vi "FinalizeHWI.vi"(8 "error in (no error)":errorcluster, 10 "Master Device in":refnum<class "Master Device.lvclass">, 11 "SRS_DS345 in":refnum<class "SRS_DS345.lvclass">) -> (0 "error out":errorcluster, 2 "Master Device out":refnum<class "Master Device.lvclass">, 3 "SRS_DS345 out":refnum<class "SRS_DS345.lvclass">)   [LabVIEW 2013, in "SRS_DS345.lvclass"]
uses:
  SRS_DS345.lvclass
  <vilib>/Utility/error.llb/DialogType.ctl
  Master Device/Master Device.lvclass
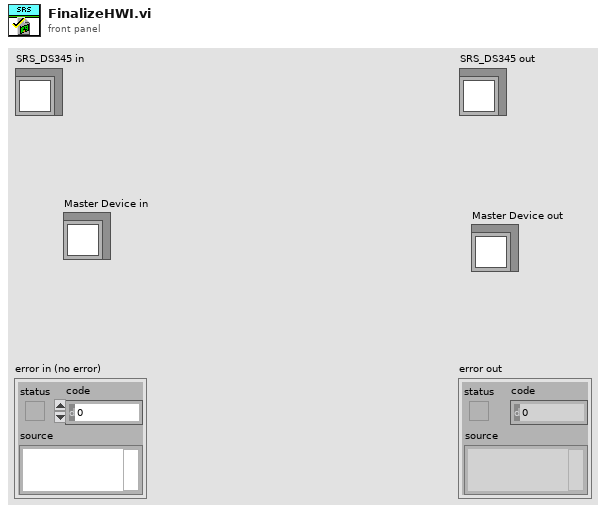
[diagram p1: front panel]
types:
  T1 = typedef "DialogType.ctl" = u16
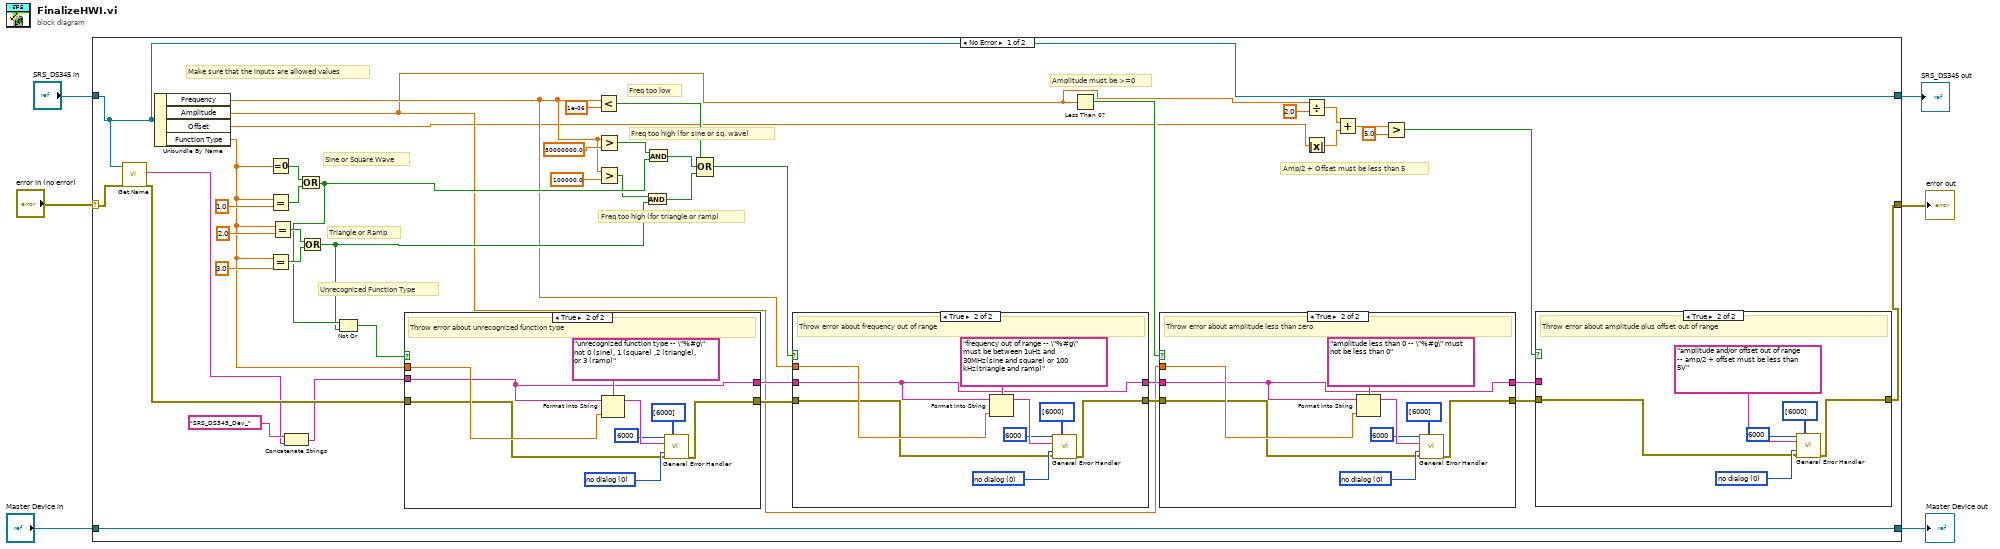
[diagram p0: block diagram]
diagram:
  n1 = case shown="No Error" "error in (no error)" {
    selector: "error in (no error)" -> [w42 w93]
    tunnel: [w8 w93] -> w5
    tunnel: [w9 w92] -> w3
    tunnel: "Master Device in" -> [w9 w92]
    tunnel: "SRS_DS345 in" -> [w7 w91]
    tunnel: [w7 w91] -> w1
    frame No Error {
      # "Amp/2 + Offset must be less than 5"
      # "Amplitude must be >=0"
      # "Freq too high (for triangle or ramp)"
      # "Freq too high (for sine or sq. wave)"
      # "Freq too low"
      # "Unrecognized Function Type"
      # "Triangle or Ramp"
      # "Sine or Square Wave"
      # "Make sure that the inputs are allowed values"
      n2 = call-dynamic "Get Name.vi"("error in (no error)"=w42, "Device in"=w7) -> ("error out"=w41:errorcluster, "Name"=w26:string)  [unwired: 7 in, 1 out]
      n3 = Unbundle By Name(w7) -> ("Frequency"=w23:dbl, "Amplitude"=w19:dbl, "Offset"=w17:dbl, "Function Type"=w40:dbl)
      n4 = Equal To 0?(x=w40) -> (x = 0?=w48:bool)
      n5 = Equal?(x=w40, y=1.0) -> (x = y?=w49:bool)
      n6 = Equal?(x=w40, y=3.0) -> (x = y?=w45:bool)
      n7 = Equal?(x=w40, y=2.0) -> (x = y?=w44:bool)
      n8 = Concatenate Strings("SRS_DS345_Dev_", w26) -> (w25:string)
      n9 = Or(x=w48, y=w49) -> (x .or. y?=w35:bool)
      n10 = Or(x=w44, y=w45) -> (x .or. y?=w33:bool)
      n11 = Not Or(1:w33, 2:w35) -> (0:w43:bool)
      n12 = case shown="True" w43 {
        tunnel: w41 -> [w81 w86]
        tunnel: w25 -> [w80 w82]
        tunnel: w40 -> [_ w89]
        tunnel: [w81 w83] -> w28
        tunnel: [w80 w82] -> w24
        frame False {
        }
        frame True {
          w87 = T1 0 items=["no dialog", "OK message", "continue or stop message", "OK message + warnings", "continue/stop + warnings"] ("type of dialog (OK msg:1)")
          # "Throw error about unrecognized function type"
          n13 = Format Into String(format string="unrecognized function type -- \"%#g\" not 0 (sine), 1 (square) ,2 (triangle), or 3 (ramp)", initial string=w82, w89) -> (resulting string=w88:string)  [unwired: 1 in, 1 out]
          n14 = call <vilib>:"General Error Handler.vi"("[error code] (0)"=6000 ("error code (no error:0)"), "[user-defined codes]"=i32[] [6000], "[error source] (\" \")"=w88, "type of dialog (OK msg:1)"=w87, "error in (no error)"=w86) -> ("error out"=w83:errorcluster)  [unwired: 6 in, 4 out]
        }
      }
      n15 = Less?(x=w23, y=1e-06) -> (x < y?=w30:bool)
      n16 = Greater?(x=w23, y=30000000.0) -> (0:w36:bool)
      n17 = Greater?(x=w23, y=100000.0) -> (0:w34:bool)
      n18 = And(x=w34, y=w33) -> (x .and. y?=w32:bool)
      n19 = And(x=w36, y=w35) -> (x .and. y?=w31:bool)
      n20 = Compound Arithmetic op=OR(w30, w31, w32) -> (w29:bool)
      n21 = case shown="True" w29 {
        tunnel: w28 -> [w70 w75]
        tunnel: w23 -> [_ w78]
        tunnel: [w70 w72] -> w20
        tunnel: w24 -> [w69 w71]
        tunnel: [w69 w71] -> w21
        frame False {
        }
        frame True {
          w76 = T1 0 items=["no dialog", "OK message", "continue or stop message", "OK message + warnings", "continue/stop + warnings"] ("type of dialog (OK msg:1)")
          # "Throw error about frequency out of range"
          n22 = Format Into String(format string="frequency out of range -- \"%#g\" must be between 1uHz and 30MHz(sine and square) or 100 kHz(triangle and ramp)", initial string=w71, w78) -> (resulting string=w77:string)  [unwired: 1 in, 1 out]
          n23 = call <vilib>:"General Error Handler.vi"("[error code] (0)"=6000 ("error code (no error:0)"), "[user-defined codes]"=i32[] [6000], "[error source] (\" \")"=w77, "type of dialog (OK msg:1)"=w76, "error in (no error)"=w75) -> ("error out"=w72:errorcluster)  [unwired: 6 in, 4 out]
        }
      }
      n24 = Less Than 0?(x=w19) -> (x < 0?=w22:bool)
      n25 = case shown="True" w22 {
        tunnel: w20 -> [w59 w64]
        tunnel: w19 -> [_ w67]
        tunnel: [w59 w61] -> w11
        tunnel: w21 -> [w58 w60]
        tunnel: [w58 w60] -> w12
        frame False {
        }
        frame True {
          w65 = T1 0 items=["no dialog", "OK message", "continue or stop message", "OK message + warnings", "continue/stop + warnings"] ("type of dialog (OK msg:1)")
          # "Throw error about amplitude less than zero"
          n26 = Format Into String(format string="amplitude less than 0 -- \"%#g\" must not be less than 0", initial string=w60, w67) -> (resulting string=w66:string)  [unwired: 1 in, 1 out]
          n27 = call <vilib>:"General Error Handler.vi"("[error code] (0)"=6000 ("error code (no error:0)"), "[user-defined codes]"=i32[] [6000], "[error source] (\" \")"=w66, "type of dialog (OK msg:1)"=w65, "error in (no error)"=w64) -> ("error out"=w61:errorcluster)  [unwired: 6 in, 4 out]
        }
      }
      n28 = Divide(x=w19, y=2.0) -> (x/y=w16:dbl)
      n29 = Absolute Value(x=w17) -> (abs(x)=w15:dbl)
      n30 = Add(x=w16, y=w15) -> (x+y=w14:dbl)
      n31 = Greater?(x=w14, y=5.0) -> (0:w10:bool)
      n32 = case shown="True" w10 {
        tunnel: w11 -> [w51 w56]
        tunnel: [w51 w53] -> w8
        tunnel: w12 -> [_ _]
        frame False {
        }
        frame True {
          w57 = T1 0 items=["no dialog", "OK message", "continue or stop message", "OK message + warnings", "continue/stop + warnings"] ("type of dialog (OK msg:1)")
          # "Throw error about amplitude plus offset out of range"
          n33 = call <vilib>:"General Error Handler.vi"("[error code] (0)"=6000 ("error code (no error:0)"), "[user-defined codes]"=i32[] [6000], "[error source] (\" \")"="amplitude and/or offset out of range -- amp/2 + offset must be less than 5V" ("format string"), "type of dialog (OK msg:1)"=w57, "error in (no error)"=w56) -> ("error out"=w53:errorcluster)  [unwired: 6 in, 4 out]
        }
      }
    }
    frame Error {
    }
  }
  "error out" <- w5
  "SRS_DS345 out" <- w1
  "Master Device out" <- w3
